vi "CSM - Post Message.vi"(7 "Current Module (\"\" to Generate an ID)":string, 8 "Error In (No Error)":errorcluster, 9 "Target Module":string="Target", 10 "Arguments (\"\")":string, 11 "State":string="API State") -> (0 "error out":errorcluster)   [LabVIEW 2017, in "Communicable State Machine.lvlib"]
doc: "Sends an asynchronous message to the specified CSM module. Since the transmission is asynchronous, this VI does not wait for a reply, and code execution continues immediately after the message is sent. If the CSM module does not exist, a \"Target Error\" is returned.\n\n> ![NOTE] \n>\n> Asynchronous messages sent using this VI are strictly asynchronous without return. Return arguments from asynchronous messages cannot be retrieved.\n\n> [!NOTE] \n> <b>Asynchronous Message</b>\n>\n> An Asynchronous Message is a type of message. After a CSM sends an asynchronous message, it immediately continues to execute subsequent code without waiting for the callee to complete message processing. Asynchronous messages are divided into Asynchronous Call (`->`) and Asynchronous Call without Reply (`->|`). The only difference is that with an Asynchronous Call without Reply (`->|`), the callee will not return the result to the caller after completing the operation.\n>\n> <b>Errors occurring at the Caller:</b>\n>\n> - If the input target module is `\"\"`, a `NO Target Error` is generated.\n> - If the input module does not exist, a `Target Error` is generated.\n>\n> <b>Caller does not wait for return:</b>\n>\n> - If the caller is a CSM module, it enters the \"Async Message Posted\" state after sending the message in the Parse State Queue++ VI.\n> - If it is an API call, it continues to execute subsequent code. The API can only send Asynchronous without Reply messages.\n>\n> <b>Return:</b>\n>\n> - <b>If the caller is a CSM module:</b>\n> - Normally, it enters the \"Async Response\" state to handle the return. If an error occurs at the callee, this information is still the result of the message. It is handled in the \"Async Response\" state, and this error information can be obtained from Additional Information.\n> - If an error occurs at the caller, it causes the CSM state machine to enter the \"Error Handler\" module to handle the error.\n> - There is no return if the API can only send Asynchronous without Reply messages.\n\n> [!NOTE] \n> <b>CSM Message Target Module Description</b>\n>\n> In Normal Mode, the target module for a CSM message is the specified module name. System-level modules start with a `.` in their name. The target module for a CSM message includes the `.` in the name. For example, if the requested module name is `.System`, the target module for the CSM message is `.System`. In Worker Mode, the target module for a CSM message can only be the overall module name, not the node name. For example, if the requested module name is `Worker#`, the target module for the CSM message is `Worker`. In Chain of Responsibility Mode, the target module for a CSM message can only be the overall module name, not the node name. For example, if the requested module name is `Chain$1`, the target module for the CSM message is `Chain`.\n\n\n-- <b>Controls</b> --\n- <b>Current Module (\"\" to Generate an ID)</b>: Name of the current module. If empty, a temporary ID is generated for debugging purposes to identify the location.\n- <b>State</b>: Message string.\n- <b>Arguments (\"\")</b>: Message arguments.\n- <b>Target Module</b>: Name of the target module."
uses:
  Communicable State Machine.lvlib
  _Support/Typedef/_CSM_MSG_TYPE.ctl
  CSM - Message Type.ctl
  _Support/CSMQ/_CSMObj-Message Check.vi
  _Support/CSMQ/_CSMObj-Enqueue Cross-Module Message.vi
  _Support/CSMQ/_CSMOFGV Get.vi
  _Support/GlobalEvent/GEvt-Convert Filter Rules - v1.0.vi
  _Support/ChangeFlag/FlagInstance-GEvt Filter.vi
  _Support/GlobalEvent/GEvt-Generate with Rule Check.vi
  _Shared/CSM - System States.vi
  _Support/Priority Queue/Enqueue Element.vi
  _Support/ChangeFlag/ChangeFlag-Read.vi
  _Support/GlobalEvent/LogFilter/LogFilter - Check.vi
  _Support/GlobalEvent/LogFilter/SettingVIs/Set CSM StateType Filter.vi
  _Support/GlobalEvent/LogFilter/SettingVIs/Set Global StateType Filter.vi
  _Support/GlobalEvent/LogFilter/SettingVIs/Set CSM State Filter.vi
  _Support/GlobalEvent/LogFilter/SettingVIs/Set CSM LogType Filter.vi
  _Support/GlobalEvent/LogFilter/SettingVIs/Set Global State Filter.vi
  _Support/GlobalEvent/LogFilter/SettingVIs/Set Global LogType Filter.vi
  _Support/GlobalEvent/LogFilter/SettingVIs/Set Global CSM Filter.vi
  _Support/GlobalEvent/FGV-GEvt Filter Rules(lvlibp).vi
  _Support/ChangeFlag/ChangeFlagDB.vi
  _Support/Error/CSM Not Allowed Message.vi
  _Support/CSMQ/_CSMOFGV(lvlibp).vi
  _Support/GlobalEvent/LogFilter/LogFilter.lvclass
  _Shared/CSM Shared.lvlib
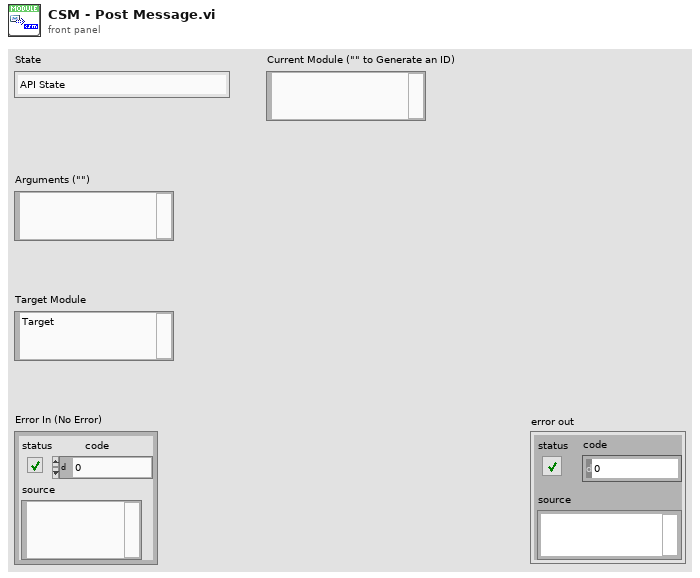
[diagram p1: front panel]
types:
  T1 = typedef "Communicable State Machine.lvlib/_CSM_MSG_TYPE.ctl" = enum16{"Sync Message(-@)", "Async Message(->)", "Async without Response(->|)", "Async Response", "Broadcast(-><all>)", "Broadcast(-><status>)", "Broadcast(-><interrupt>)", "Append to JKISM States", "Append to JKISM States(High Priority)", "Broadcast(-><state>)"}
  T2 = typedef "Communicable State Machine.lvlib/CSM - Message Type.ctl" = enum16{"Async", "Async without Reply", "Sync"}
  T3 = typedef "Communicable State Machine.lvlib/GEvt-Refs.ctl" = cluster{"Event":refnum<user-event>, "Queues":refnum<queue>[], "Valid":bool}
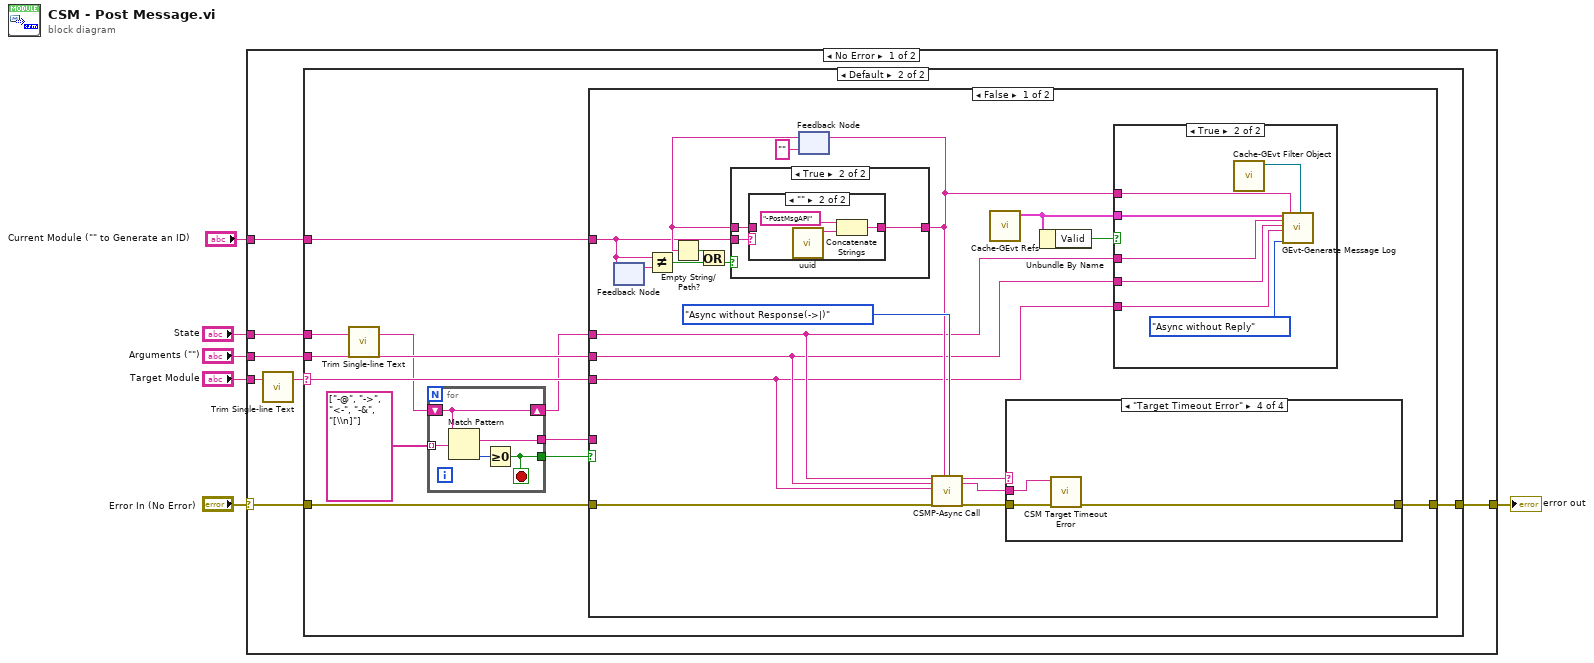
[diagram p0: block diagram]
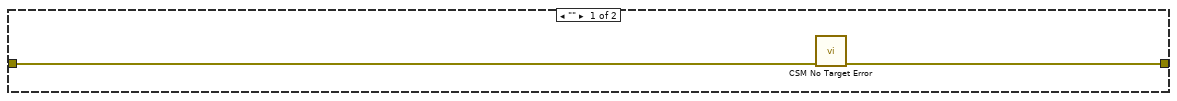
[diagram p2: hidden frame]
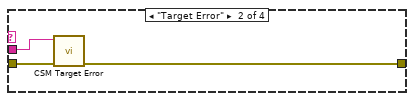
[diagram p7: hidden frame]
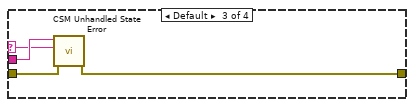
[diagram p8: hidden frame]
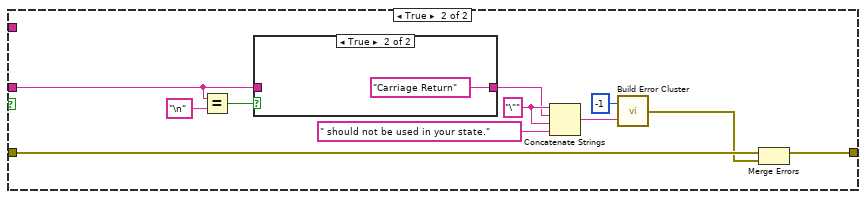
[diagram p9: hidden frame]
diagram:
  n1 = case shown="No Error" "Error In (No Error)" {
    selector: "Error In (No Error)" -> [w11 w90]
    tunnel: "State" -> [w8 _]
    tunnel: [w12 w90] -> w4
    tunnel: "Arguments (\"\")" -> [w9 _]
    tunnel: "Target Module" -> [w13 _]
    tunnel: "Current Module (\"\" to Generate an ID)" -> [w7 _]
    frame No Error {
      n2 = call "Trim Single-line Text.vi"("single-line text"=w13) -> ("trimed text"=w10:string)  [unwired: 2 in]
      n3 = case shown="Default" w10 {
        selector: w10 -> [_ w25]
        tunnel: w8 -> [_ w21]
        tunnel: w9 -> [_ w26]
        tunnel: [w14 w24] -> w12
        tunnel: w11 -> [w15 w23]
        tunnel: w7 -> [_ w16]
        frame "" {
          n4 = call "CSM No Target Error.vi"("error in (no error)"=w15) -> ("error out"=w14:errorcluster)  [unwired: 10 in]
        }
        frame Default {
          n5 = call "Trim Single-line Text.vi"("single-line text"=w21) -> ("trimed text"=w17:string)  [unwired: 2 in]
          n6 = for {
            shift-right: [w89] -> w20
            shift-left: w17 -> [w89]
            tunnel: string[] ["-@", "->", "<-", "-&", "[\\n]"] -> [w88] mode=indexing
            tunnel: [w86] -> w18
            tunnel: [w85] -> w19
            stop <- w85 stop-if-true
            n7 = Match Pattern(string=w89, regular expression=w88) -> (match substring=w86:string, offset past match=w87:i32)  [unwired: 1 in, 2 out]
            n8 = Greater Or Equal To 0?(x=w87) -> (x >= 0?=w85:bool)
          }
          n9 = case shown="False" w19 {
            tunnel: w26 -> [w28 _]
            tunnel: w25 -> [w27 _]
            tunnel: [w33 w74] -> w24
            tunnel: w23 -> [w36 w75]
            tunnel: w20 -> [w29 _]
            tunnel: w18 -> [_ w72]
            tunnel: w16 -> [w35 _]
            frame False {
              n10 = feedback #1() -> (w42:string)  [unwired: 1 in]
              n11 = feedback-in #1(w35) -> ()
              n12 = Not Equal?(x=w35, y=w42) -> (x != y?=w41:bool)
              n13 = feedback #2("") -> (w38:string)
              n14 = Empty String/Path?(string/path=w38) -> (empty?=w37:bool)
              n15 = Or(x=w37, y=w41) -> (x .or. y?=w39:bool)
              n16 = case shown="True" w39 {
                tunnel: w38 -> [w53 w56]
                tunnel: w35 -> [_ w55]
                tunnel: [w53 w54] -> w30
                frame False {
                }
                frame True {
                  n17 = case shown="\"\"" w55 {
                    selector: w55 -> [w57 _]
                    tunnel: [w57 w58] -> w54
                    tunnel: w56 -> [_ _]
                    frame Default {
                    }
                    frame "" {
                      n18 = call "uuid.vi"() -> ("UUID"=w59:string)  [unwired: 11 in]
                      n19 = Concatenate Strings("-PostMsgAPI" ("Name (\"\" to Use UUID)"), w59) -> (w58:string)
                    }
                  }
                }
              }
              n20 = feedback-in #2(w30) -> ()
              n21 = call "CSMP-Async Call.vi"("State"=w29, "Args"=w28, "Source/target"=w27, "Error In"=w36, "Module Name"=w30, "Msg Type"=_CSM_MSG_TYPE."Async without Response(->|)") -> ("State Out"=w45:string, "Args Out"=w43:string, "Error"=w44:errorcluster)  [unwired: 8 in, 3 out]
              n22 = call "Cache-GEvt Refs.vi"() -> ("CSM Global Log Ref"=w32:T3)  [unwired: 10 in, 1 out]
              n23 = case shown="\"Target Timeout Error\"" w45 {
                selector: w45 -> [_ _ w65 _]
                tunnel: w44 -> [w61 w63 w67 w70]
                tunnel: [w61 w62 w66 w69] -> w33
                tunnel: w43 -> [_ w64 w68 w71]
                frame "Async Message Posted" {
                }
                frame "Target Error" {
                  n24 = call "CSM Target Error.vi"("error in (no error)"=w63, "Arguments (As CSM Name)"=w64) -> ("error out"=w62:errorcluster)  [unwired: 9 in]
                }
                frame Default {
                  n25 = call "CSM Unhandled State Error.vi"("error in (no error)"=w67, "Undefined State"=w65, "CSM Name"=w68) -> ("error out"=w66:errorcluster)  [unwired: 8 in]
                }
                frame "Target Timeout Error" {
                  n26 = call "CSM Target Timeout Error.vi"("error in (no error)"=w70, "Arguments (As CSM Name)"=w71) -> ("error out"=w69:errorcluster)  [unwired: 9 in]
                }
              }
              n27 = Unbundle By Name(w32) -> ("Valid"=w31:bool)
              n28 = case shown="True" w31 {
                tunnel: w32 -> [_ w51]
                tunnel: w30 -> [_ w50]
                tunnel: w29 -> [_ w49]
                tunnel: w28 -> [_ w48]
                tunnel: w27 -> [_ w47]
                frame False {
                }
                frame True {
                  n29 = call "Cache-GEvt Filter Object.vi"() -> ("CSM:LogFilter.lvclass"=w52:refnum<class "LogFilter.lvclass">)  [unwired: 11 in]
                  n30 = call "GEvt-Generate Message Log.vi"("CSM Global Log Event"=w51, "Current State"=w49, "Arguments"=w48, "Source Module"=w47, "Type"=CSM_-_Message_Type."Async without Reply", "Name (\"\" to Use UUID)"=w50, "CSM:LogFilter.lvclass"=w52) -> ()  [unwired: 11 in, 2 out]
                }
              }
            }
            frame True {
              w79 = "\"" ("string")
              n31 = Equal?(x=w72, y="\n" ("regular expression")) -> (x = y?=w76:bool)
              n32 = case shown="True" w76 {
                tunnel: [w83 "Carriage Return" ("State")] -> w78
                tunnel: w72 -> [w83 _]
                frame False {
                }
                frame True {
                }
              }
              n33 = Concatenate Strings(w79, w78, w79, " should not be used in your state." ("String to Prepend to source (\"\")")) -> (w80:string)
              n34 = call "Build Error Cluster.vi"("String to Prepend to Source (\"\")"=w80, "Code"=-1 ("code")) -> ("error out"=w73:errorcluster)
              n35 = Merge Errors(w75, w73) -> (w74:errorcluster)
            }
          }
        }
      }
    }
    frame Error {
    }
  }
  "error out" <- w4
